vi "SetVersionInformationOnProject.vi"(7 "Project ref":refnum<vi>, 8 "error in (no error)":errorcluster, 11 "ProjectItem in":refnum<class "ProjectItem.lvclass">) -> (0 "error out":errorcluster, 3 "ProjectItem out":refnum<class "ProjectItem.lvclass">)   [LabVIEW 2019, in "SolutionBuilder.lvlib" / "ProjectItem.lvclass"]
uses:
  ProjectItem.lvclass
  Community/slnbld_BuildSpecVersion.ctl
  ProjectItem.lvclass/ProjectItem.ctl
  <vilib>/AppBuilder/AB_API_Simple/Build Specification Version.ctl
  <vilib>/AppBuilder/AB_API_Simple/NI_App_Builder_API.lvlib
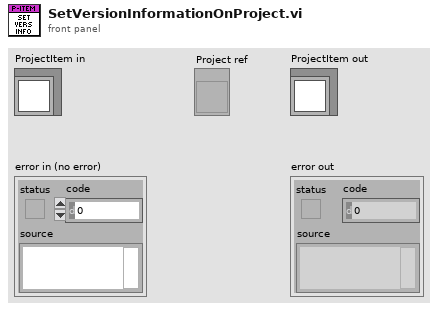
[diagram p1: front panel]
types:
  T1 = typedef "SolutionBuilder.lvlib/ProjectItem.lvclass/slnbld_BuildSpecVersion.ctl" = cluster{"Major":u16, "Minor":u16, "Fix":u16, "Build":u16}
  T2 = typedef "NI_App_Builder_API.lvlib/Build Specification Version.ctl" = cluster{"Major":u16, "Minor":u16, "Fix":u16, "Build":u16}
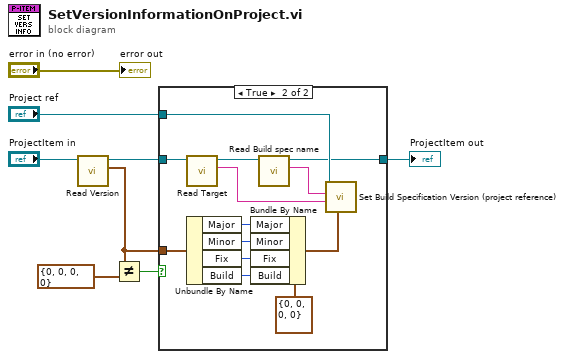
[diagram p0: block diagram]
diagram:
  n1 = call "Read Version.vi"("ProjectItem in"="ProjectItem in") -> ("Version"=w3:T1, "ProjectItem out"=w5:refnum<class "ProjectItem.lvclass">)  [unwired: 8 in, 1 out]
  n2 = Not Equal?(x=w3, y=T1 {"Major"=0, "Minor"=0, "Fix"=0, "Build"=0}) -> (x != y?=w1:bool)
  n3 = case shown="True" w1 {
    tunnel: "Project ref" -> [_ w17]
    tunnel: w5 -> [w9 w15]
    tunnel: [w9 w12] -> w4
    tunnel: w3 -> [_ w10]
    frame False {
    }
    frame True {
      n4 = call "Read Target.vi"("ProjectItem in"=w15) -> ("Target"=w16:string, "ProjectItem out"=w14:refnum<class "ProjectItem.lvclass">)  [unwired: 9 in]
      n5 = Unbundle By Name(w10) -> ("Major"=w22:u16, "Minor"=w21:u16, "Fix"=w20:u16, "Build"=w19:u16)
      n6 = Bundle By Name(cluster=T2 {"Major"=0, "Minor"=0, "Fix"=0, "Build"=0} ("Build Specification Version"), "Major"=w22, "Minor"=w21, "Fix"=w20, "Build"=w19) -> (w11:T2)
      n7 = call "Read Build spec name.vi"("ProjectItem in"=w14) -> ("Build spec name"=w13:string, "ProjectItem out"=w12:refnum<class "ProjectItem.lvclass">)  [unwired: 9 in]
      n8 = call <vilib>:"Set Build Specification Version (project reference).vi"("Build Specification Version"=w11, "Name of target (My Computer)"=w16, "Name of build specification"=w13, "Project reference"=w17) -> ()  [unwired: 6 in, 2 out]
    }
  }
  "ProjectItem out" <- w4
  "error out" <- "error in (no error)"
